vi "sweep(SubVI).vi"(0 "data":refnum<queue>, 1 "类型":enum16{"temp", "field", "position"}(ring), 5 "steps number":i32, 7 "簇":T1={"initialize"=enum."SR830", "6221"={"6221 Resource"="GPIB0::24::INSTR", "Delta status"=FALSE, "电流|RMS(A)"=0.0}, "SR830+6221"={"source"=0, "Current(A)"=0.0, "阻抗(Ohm)"=0.0, "SR830 1"=FALSE, "SR830 2"=FALSE, "SR830 3"=FALSE, "SR830 4"=FALSE, "VISA 1"="", "VISA 2"="", "VISA 3"="", "VISA 4"="", "Reserve 1"=0, "Reserve 2"=-1, "Reserve 3"=-1, "Reserve 4"=-1, "Sensitivity 1"=-1, "Sensitivity 2"=0, "Sensitivity 3"=-1, "Sensitivity 4"=-1, "量程入 1"=0, "量程入 2"=0, "量程入 3"=0, "量程入 4"=0}, "2400"={"2400"=FALSE, "VISA"=""}, "ch"={"ch"=[], "current"=[], "change?"=[], "holding current\nwhen change ch?"=FALSE}, "Instrument"={"335 Resource"="GPIB0::24::INSTR", "Input (0:A)"=0, "Instrument Type"=enum."SVSM", "quantum design"=refnum, "Heater Output (1:1)"=1, "semaphore"=refnum, "TCP master instance"=refnum, "335 Status"=refnum, "M24C Resource"="GPIB0::24::INSTR", "4G supply"="GPIB0::24::INSTR", "Temp Status 24C"=refnum, "Temp"=refnum, "9T信号"=refnum, "limit"={"Field limit"=0.0, "Field rate limit"=0.0, "Temp limit"=0.0, "Temp low limit"=0.0, "Temp rate limit "=0.0}, "4g supply status"=refnum, "vi路径"=""}, "Aborting"=refnum, "数据文件"=refnum, "warning"=refnum, "2614B"={"2614B chA"=FALSE, "2614B chB"=FALSE, "VISA"=""}} {"Instrument"."Input (0:A)" items=["A", "B"]; "Instrument"."Heater Output (1:1)" items=["1"=1, "2"=2]; "SR830+6221"."Sensitivity 4" items=["Auto Gain"=-1, "2 nV/fA"=0, "5 nV/fA"=1, "10 nV/fA"=2, "20 nV/fA"=3, "50 nV/fA"=4, "100 nV/fA"=5, "200 nV/fA"=6, "500 nV/fA"=7, "1 uV/pA"=8, "2 uV/pA"=9, "5 uV/pA"=10, "10 uV/pA"=11, "20 uV/pA"=12, "50 uV/pA"=13, "100 uV/pA"=14, "200 uV/pA"=15, "500 uV/pA"=16, "1 mV/nA"=17, "2 mV/nA"=18, "5 mV/nA"=19, "10 mV/nA"=20, "20 mV/nA"=21, "50 mV/nA"=22, "100 mV/nA"=23, "200 mV/nA"=24, "500 mV/mA"=25, "1 V/uA"=26]; "SR830+6221"."Sensitivity 3" items=["Auto Gain"=-1, "2 nV/fA"=0, "5 nV/fA"=1, "10 nV/fA"=2, "20 nV/fA"=3, "50 nV/fA"=4, "100 nV/fA"=5, "200 nV/fA"=6, "500 nV/fA"=7, "1 uV/pA"=8, "2 uV/pA"=9, "5 uV/pA"=10, "10 uV/pA"=11, "20 uV/pA"=12, "50 uV/pA"=13, "100 uV/pA"=14, "200 uV/pA"=15, "500 uV/pA"=16, "1 mV/nA"=17, "2 mV/nA"=18, "5 mV/nA"=19, "10 mV/nA"=20, "20 mV/nA"=21, "50 mV/nA"=22, "100 mV/nA"=23, "200 mV/nA"=24, "500 mV/mA"=25, "1 V/uA"=26]; "SR830+6221"."Sensitivity 1" items=["Auto Gain"=-1, "2 nV/fA"=0, "5 nV/fA"=1, "10 nV/fA"=2, "20 nV/fA"=3, "50 nV/fA"=4, "100 nV/fA"=5, "200 nV/fA"=6, "500 nV/fA"=7, "1 uV/pA"=8, "2 uV/pA"=9, "5 uV/pA"=10, "10 uV/pA"=11, "20 uV/pA"=12, "50 uV/pA"=13, "100 uV/pA"=14, "200 uV/pA"=15, "500 uV/pA"=16, "1 mV/nA"=17, "2 mV/nA"=18, "5 mV/nA"=19, "10 mV/nA"=20, "20 mV/nA"=21, "50 mV/nA"=22, "100 mV/nA"=23, "200 mV/nA"=24, "500 mV/mA"=25, "1 V/uA"=26]; "SR830+6221"."Sensitivity 2" items=["Auto Gain"=-1, "2 nV/fA"=0, "5 nV/fA"=1, "10 nV/fA"=2, "20 nV/fA"=3, "50 nV/fA"=4, "100 nV/fA"=5, "200 nV/fA"=6, "500 nV/fA"=7, "1 uV/pA"=8, "2 uV/pA"=9, "5 uV/pA"=10, "10 uV/pA"=11, "20 uV/pA"=12, "50 uV/pA"=13, "100 uV/pA"=14, "200 uV/pA"=15, "500 uV/pA"=16, "1 mV/nA"=17, "2 mV/nA"=18, "5 mV/nA"=19, "10 mV/nA"=20, "20 mV/nA"=21, "50 mV/nA"=22, "100 mV/nA"=23, "200 mV/nA"=24, "500 mV/mA"=25, "1 V/uA"=26]; "SR830+6221"."Reserve 4" items=["Auto Gain"=-1, "2 nV/fA"=0, "5 nV/fA"=1, "10 nV/fA"=2, "20 nV/fA"=3, "50 nV/fA"=4, "100 nV/fA"=5, "200 nV/fA"=6, "500 nV/fA"=7, "1 uV/pA"=8, "2 uV/pA"=9, "5 uV/pA"=10, "10 uV/pA"=11, "20 uV/pA"=12, "50 uV/pA"=13, "100 uV/pA"=14, "200 uV/pA"=15, "500 uV/pA"=16, "1 mV/nA"=17, "2 mV/nA"=18, "5 mV/nA"=19, "10 mV/nA"=20, "20 mV/nA"=21, "50 mV/nA"=22, "100 mV/nA"=23, "200 mV/nA"=24, "500 mV/mA"=25, "1 V/uA"=26]; "SR830+6221"."Reserve 3" items=["Auto Reserve"=-1, "High Reserve"=0, "Normal"=1, "Low Noise"=2]; "SR830+6221"."Reserve 2" items=["Auto Reserve"=-1, "High Reserve"=0, "Normal"=1, "Low Noise"=2]; "SR830+6221"."Reserve 1" items=["Auto Reserve"=-1, "High Reserve"=0, "Normal"=1, "Low Noise"=2]; "SR830+6221"."source" items=["SR830 1", "SR830 2", "SR830 3", "SR830 4"]}, 9 "Field":dbl=300.0, 11 "Mode":i32(ring) items=["Persistent", "Driven"], 13 "Field 2":dbl=300.0, 14 "Rate、speed":dbl=10.0) -> (4 "输出簇":T1={"initialize"=enum."SR830", "6221"={"6221 Resource"="GPIB0::24::INSTR", "Delta status"=FALSE, "电流|RMS(A)"=0.0}, "SR830+6221"={"source"=0, "Current(A)"=0.0, "阻抗(Ohm)"=0.0, "SR830 1"=FALSE, "SR830 2"=FALSE, "SR830 3"=FALSE, "SR830 4"=FALSE, "VISA 1"="", "VISA 2"="", "VISA 3"="", "VISA 4"="", "Reserve 1"=0, "Reserve 2"=-1, "Reserve 3"=-1, "Reserve 4"=-1, "Sensitivity 1"=-1, "Sensitivity 2"=0, "Sensitivity 3"=-1, "Sensitivity 4"=-1, "量程入 1"=0, "量程入 2"=0, "量程入 3"=0, "量程入 4"=0}, "2400"={"2400"=FALSE, "VISA"=""}, "ch"={"ch"=[], "current"=[], "change?"=[], "holding current\nwhen change ch?"=FALSE}, "Instrument"={"335 Resource"="GPIB0::24::INSTR", "Input (0:A)"=0, "Instrument Type"=enum."SVSM", "quantum design"=refnum, "Heater Output (1:1)"=1, "semaphore"=refnum, "TCP master instance"=refnum, "335 Status"=refnum, "M24C Resource"="GPIB0::24::INSTR", "4G supply"="GPIB0::24::INSTR", "Temp Status 24C"=refnum, "Temp"=refnum, "9T信号"=refnum, "limit"={"Field limit"=0.0, "Field rate limit"=0.0, "Temp limit"=0.0, "Temp low limit"=0.0, "Temp rate limit "=0.0}, "4g supply status"=refnum, "vi路径"=""}, "Aborting"=refnum, "数据文件"=refnum, "warning"=refnum, "2614B"={"2614B chA"=FALSE, "2614B chB"=FALSE, "VISA"=""}} {"Instrument"."Input (0:A)" items=["A", "B"]; "Instrument"."Heater Output (1:1)" items=["1"=1, "2"=2]; "SR830+6221"."Sensitivity 4" items=["Auto Gain"=-1, "2 nV/fA"=0, "5 nV/fA"=1, "10 nV/fA"=2, "20 nV/fA"=3, "50 nV/fA"=4, "100 nV/fA"=5, "200 nV/fA"=6, "500 nV/fA"=7, "1 uV/pA"=8, "2 uV/pA"=9, "5 uV/pA"=10, "10 uV/pA"=11, "20 uV/pA"=12, "50 uV/pA"=13, "100 uV/pA"=14, "200 uV/pA"=15, "500 uV/pA"=16, "1 mV/nA"=17, "2 mV/nA"=18, "5 mV/nA"=19, "10 mV/nA"=20, "20 mV/nA"=21, "50 mV/nA"=22, "100 mV/nA"=23, "200 mV/nA"=24, "500 mV/mA"=25, "1 V/uA"=26]; "SR830+6221"."Sensitivity 3" items=["Auto Gain"=-1, "2 nV/fA"=0, "5 nV/fA"=1, "10 nV/fA"=2, "20 nV/fA"=3, "50 nV/fA"=4, "100 nV/fA"=5, "200 nV/fA"=6, "500 nV/fA"=7, "1 uV/pA"=8, "2 uV/pA"=9, "5 uV/pA"=10, "10 uV/pA"=11, "20 uV/pA"=12, "50 uV/pA"=13, "100 uV/pA"=14, "200 uV/pA"=15, "500 uV/pA"=16, "1 mV/nA"=17, "2 mV/nA"=18, "5 mV/nA"=19, "10 mV/nA"=20, "20 mV/nA"=21, "50 mV/nA"=22, "100 mV/nA"=23, "200 mV/nA"=24, "500 mV/mA"=25, "1 V/uA"=26]; "SR830+6221"."Sensitivity 1" items=["Auto Gain"=-1, "2 nV/fA"=0, "5 nV/fA"=1, "10 nV/fA"=2, "20 nV/fA"=3, "50 nV/fA"=4, "100 nV/fA"=5, "200 nV/fA"=6, "500 nV/fA"=7, "1 uV/pA"=8, "2 uV/pA"=9, "5 uV/pA"=10, "10 uV/pA"=11, "20 uV/pA"=12, "50 uV/pA"=13, "100 uV/pA"=14, "200 uV/pA"=15, "500 uV/pA"=16, "1 mV/nA"=17, "2 mV/nA"=18, "5 mV/nA"=19, "10 mV/nA"=20, "20 mV/nA"=21, "50 mV/nA"=22, "100 mV/nA"=23, "200 mV/nA"=24, "500 mV/mA"=25, "1 V/uA"=26]; "SR830+6221"."Sensitivity 2" items=["Auto Gain"=-1, "2 nV/fA"=0, "5 nV/fA"=1, "10 nV/fA"=2, "20 nV/fA"=3, "50 nV/fA"=4, "100 nV/fA"=5, "200 nV/fA"=6, "500 nV/fA"=7, "1 uV/pA"=8, "2 uV/pA"=9, "5 uV/pA"=10, "10 uV/pA"=11, "20 uV/pA"=12, "50 uV/pA"=13, "100 uV/pA"=14, "200 uV/pA"=15, "500 uV/pA"=16, "1 mV/nA"=17, "2 mV/nA"=18, "5 mV/nA"=19, "10 mV/nA"=20, "20 mV/nA"=21, "50 mV/nA"=22, "100 mV/nA"=23, "200 mV/nA"=24, "500 mV/mA"=25, "1 V/uA"=26]; "SR830+6221"."Reserve 4" items=["Auto Gain"=-1, "2 nV/fA"=0, "5 nV/fA"=1, "10 nV/fA"=2, "20 nV/fA"=3, "50 nV/fA"=4, "100 nV/fA"=5, "200 nV/fA"=6, "500 nV/fA"=7, "1 uV/pA"=8, "2 uV/pA"=9, "5 uV/pA"=10, "10 uV/pA"=11, "20 uV/pA"=12, "50 uV/pA"=13, "100 uV/pA"=14, "200 uV/pA"=15, "500 uV/pA"=16, "1 mV/nA"=17, "2 mV/nA"=18, "5 mV/nA"=19, "10 mV/nA"=20, "20 mV/nA"=21, "50 mV/nA"=22, "100 mV/nA"=23, "200 mV/nA"=24, "500 mV/mA"=25, "1 V/uA"=26]; "SR830+6221"."Reserve 3" items=["Auto Reserve"=-1, "High Reserve"=0, "Normal"=1, "Low Noise"=2]; "SR830+6221"."Reserve 2" items=["Auto Reserve"=-1, "High Reserve"=0, "Normal"=1, "Low Noise"=2]; "SR830+6221"."Reserve 1" items=["Auto Reserve"=-1, "High Reserve"=0, "Normal"=1, "Low Noise"=2]; "SR830+6221"."source" items=["SR830 1", "SR830 2", "SR830 3", "SR830 4"]}, 8 "错误输出":errorcluster)   [LabVIEW 2019, in "Scan.lvlib"]
uses:
  Scan.lvlib
  ctl/config.ctl
  <vilib>/NI/Modbus Library/API/Master/Modbus Master.lvclass
  ctl/initialize.ctl
  ctl/Instrument.ctl
  ctl/Instrument Type.ctl
  lib/QDInstrument.dll
  ctl/335 state.ctl
  ctl/limit.ctl
  ctl/9T mag field stauts.ctl
  ctl/warning.ctl
  SubVI.lvlib
  User lib.lvlib
  Get value.lvlib
  9T cmag.lvlib
panel:
  out "Field\nStatus 4":i32(ring) items=["MagnetUnknown"=0, "StablePersistent"=1, "WarmingSwitch"=2, "CoolingSwitch"=3, "StableDriven"=4, "Iterating"=5, "Charging"=6, "Discharging"=7, "CurrentError"=8, "MagnetFailure"=15]
  out "Temperature\nStatus 3":i32(ring) items=["TemperatureUnknown"=0, "Stable"=1, "Tracking"=2, "Near"=5, "Chasing"=6, "Filling"=7, "Standby"=10, "Disabled"=13, "ImpedanceNotFunction"=14, "TempFailure"=15]
  out "Temperature\nStatus":i32(ring) items=["TemperatureUnknown"=0, "Stable"=1, "Tracking"=2, "Near"=5, "Chasing"=6, "Filling"=7, "Standby"=10, "Disabled"=13, "ImpedanceNotFunction"=14, "TempFailure"=15]
  out "Field\nStatus 2":i32(ring) items=["MagnetUnknown"=0, "StablePersistent"=1, "WarmingSwitch"=2, "CoolingSwitch"=3, "StableDriven"=4, "Iterating"=5, "Charging"=6, "Discharging"=7, "CurrentError"=8, "MagnetFailure"=15]
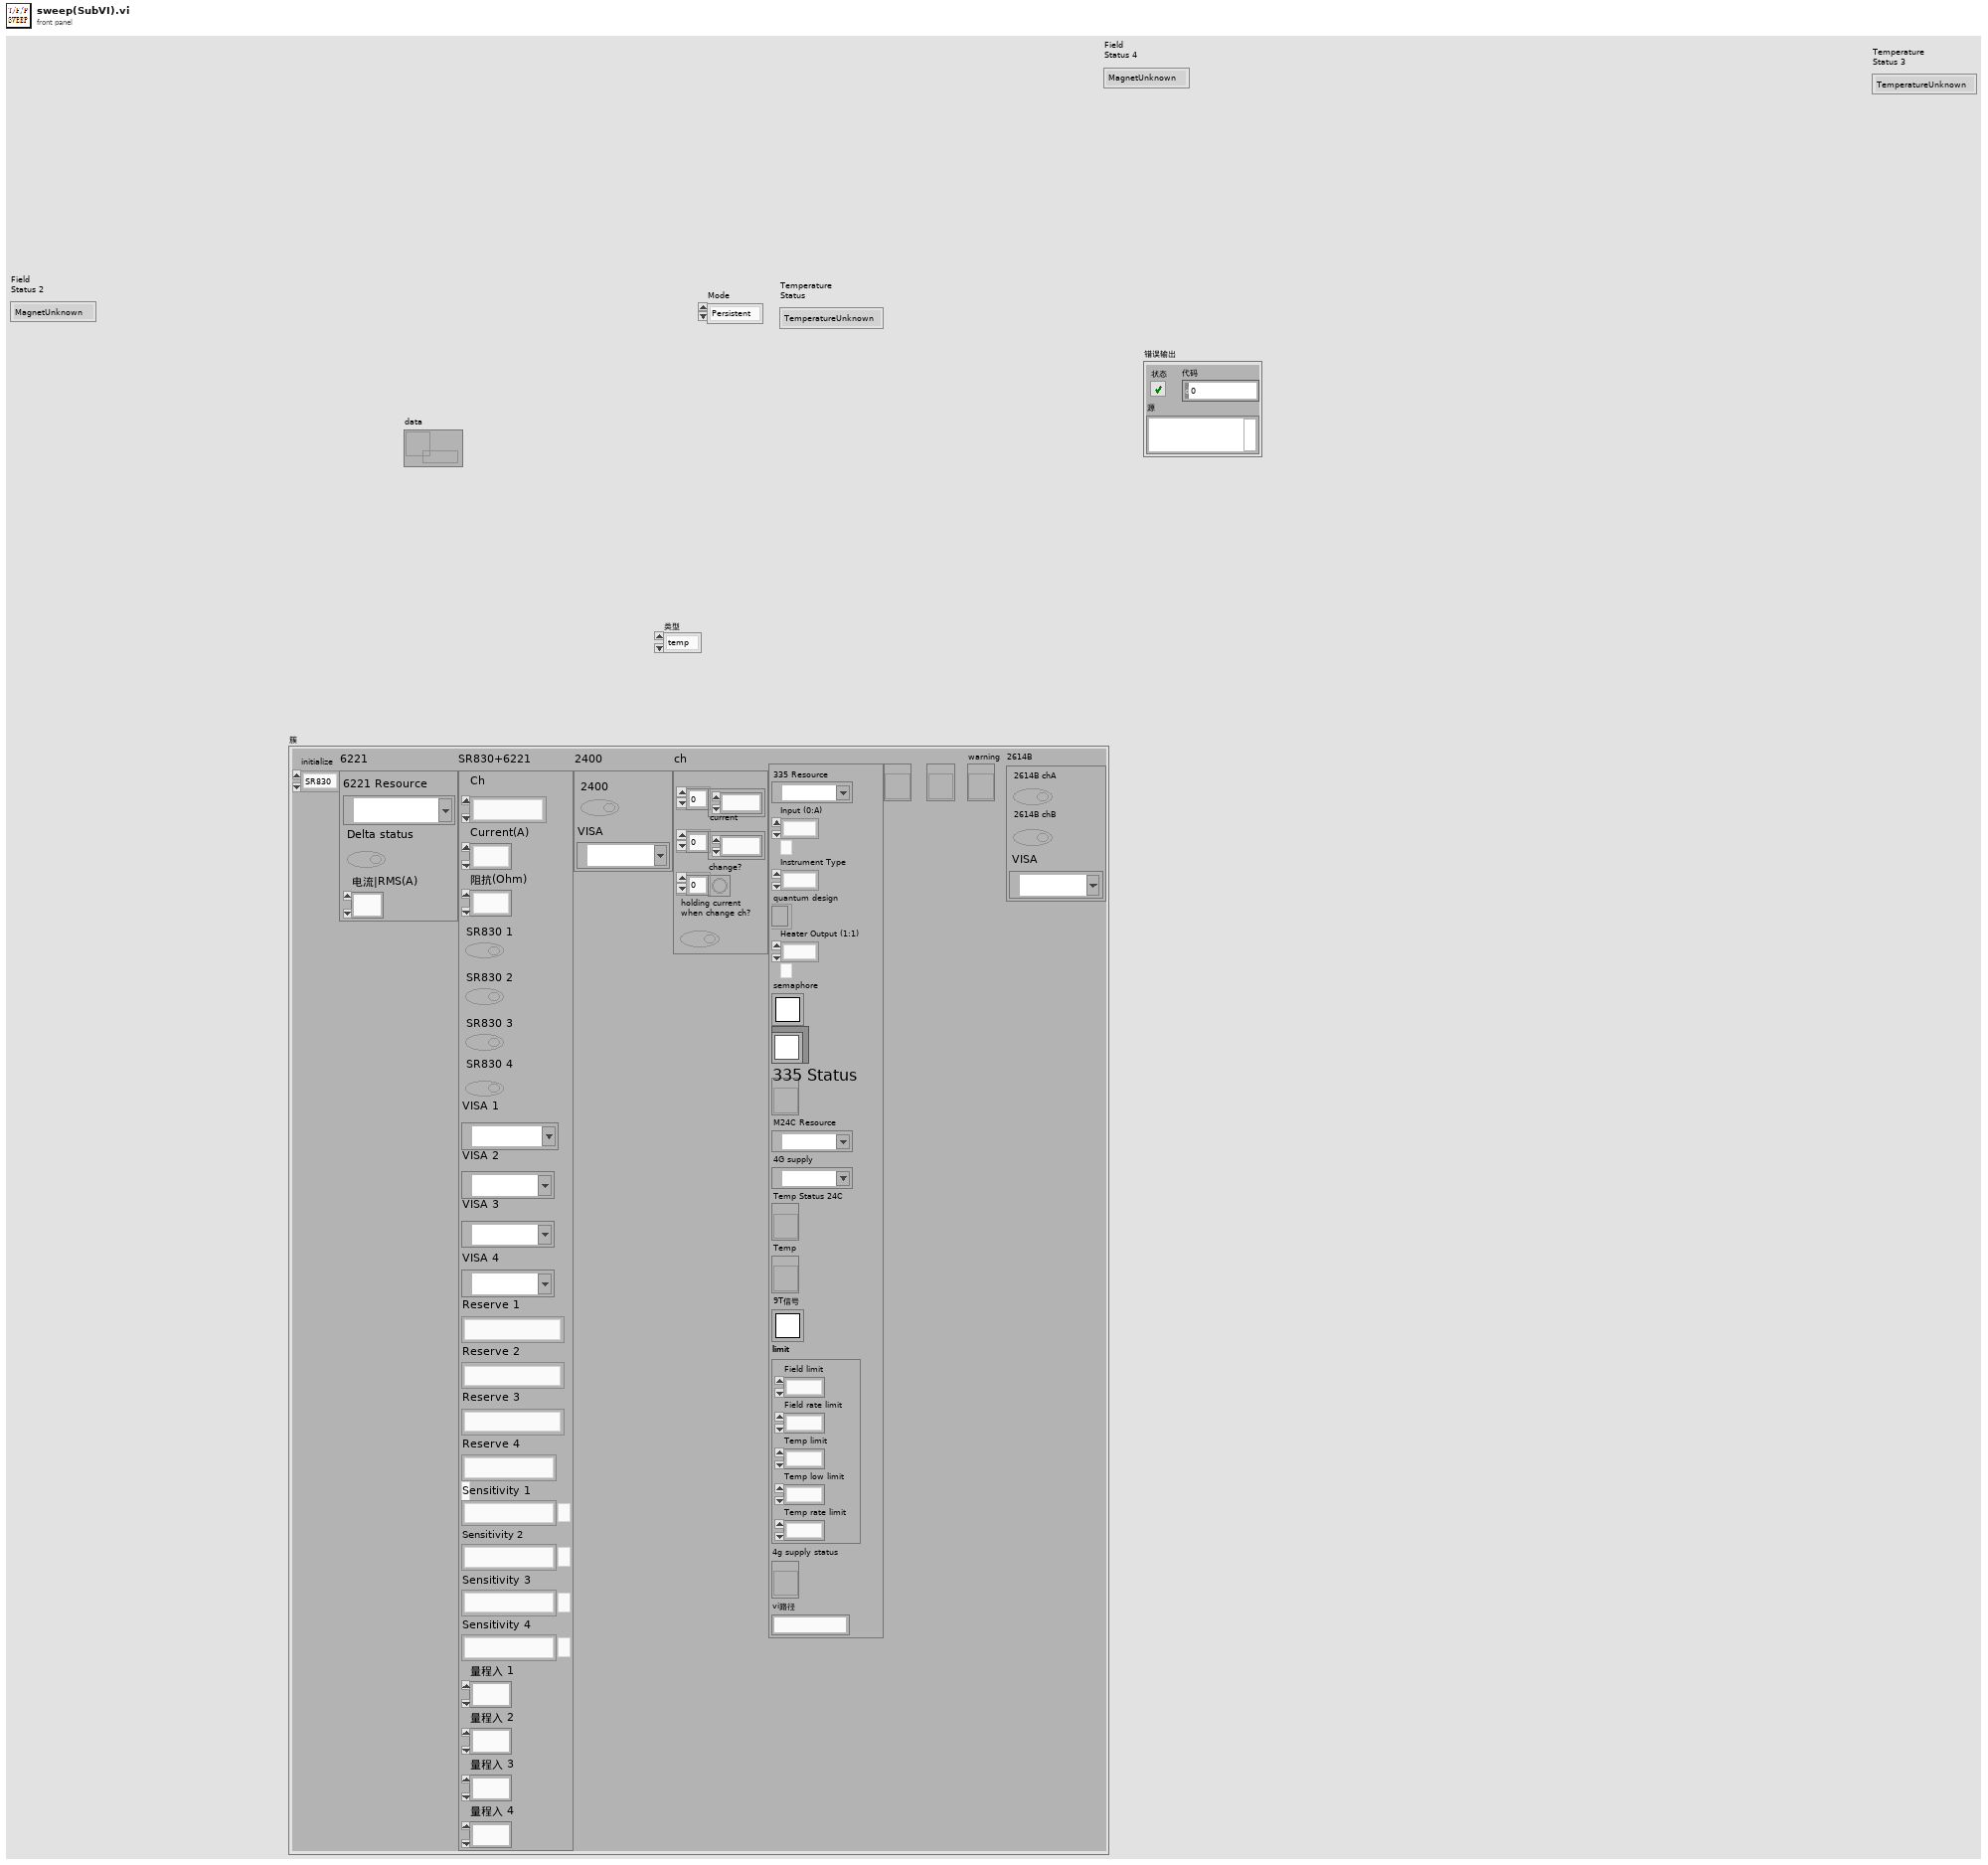
[diagram p1: front panel]
types:
  T1 = typedef "config.ctl" = cluster{"initialize":T2, "6221":cluster{"6221 Resource":refnum<visa-resource-name>, "Delta status":bool, "电流|RMS(A)":dbl}, "SR830+6221":cluster{"source":u16, "Current(A)":dbl, "阻抗(Ohm)":dbl, "SR830 1":bool, "SR830 2":bool, "SR830 3":bool, "SR830 4":bool, "VISA 1":refnum<visa-resource-name>, "VISA 2":refnum<visa-resource-name>, "VISA 3":refnum<visa-resource-name>, "VISA 4":refnum<visa-resource-name>, "Reserve 1":i16, "Reserve 2":i16, "Reserve 3":i16, "Reserve 4":i16, "Sensitivity 1":i16, "Sensitivity 2":i16, "Sensitivity 3":i16, "Sensitivity 4":i16, "量程入 1":i32, "量程入 2":i32, "量程入 3":i32, "量程入 4":i32}, "2400":cluster{"2400":bool, "VISA":refnum<visa-resource-name>}, "ch":cluster{"ch":i32[], "current":dbl[], "change?":bool[], "holding current\nwhen change ch?":bool}, "Instrument":T3, "Aborting":refnum<vi>, "数据文件":refnum<vi>, "warning":refnum<vi>, "2614B":cluster{"2614B chA":bool, "2614B chB":bool, "VISA":refnum<visa-resource-name>}}
  T2 = typedef "initialize.ctl" = enum16{"SR830", "keithley6221-SR830", "Delta", "Delta-tunnelling", "keithley6221-2182-DC"}
  T3 = typedef "Instrument.ctl" = cluster{"335 Resource":refnum<visa-resource-name>, "Input (0:A)":u16, "Instrument Type":T4, "quantum design":refnum<k24>, "Heater Output (1:1)":u16, "semaphore":T5, "TCP master instance":refnum<class "Modbus Master.lvclass">, "335 Status":refnum<vi>, "M24C Resource":refnum<visa-resource-name>, "4G supply":refnum<visa-resource-name>, "Temp Status 24C":refnum<vi>, "Temp":refnum<vi>, "9T信号":T5, "limit":T6, "4g supply status":refnum<vi>, "vi路径":string}
  T4 = typedef "Instrument Type.ctl" = enum16{"PPMS", "VersaLab", "DynaCool", "SVSM", "PPMS-Rotate", "Lakeshore335", "9T mag"}
  T5 = typedef "Semaphore RefNum" = refnum<k1>
  T6 = typedef "limit.ctl" = cluster{"Field limit":dbl, "Field rate limit":dbl, "Temp limit":dbl, "Temp low limit":dbl, "Temp rate limit ":dbl}
  T7 = typedef "335 state.ctl" = u16
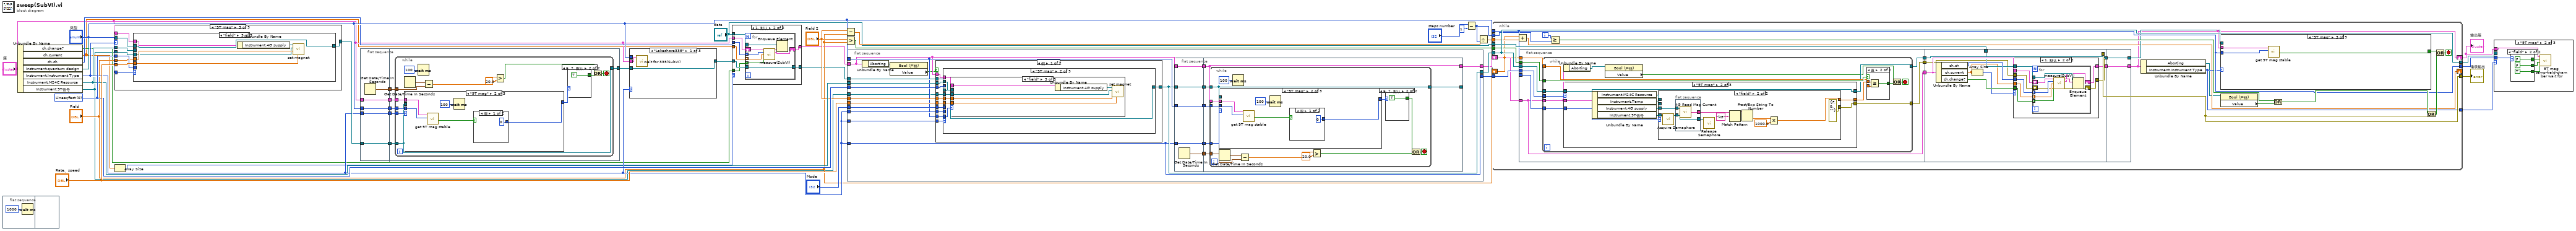
[diagram p0: block diagram]
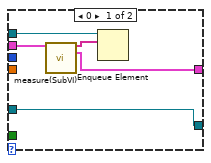
[diagram p2: hidden frame]
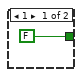
[diagram p3: hidden frame]
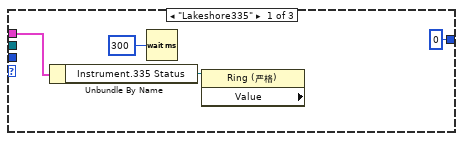
[diagram p4: hidden frame]
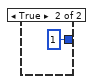
[diagram p5: hidden frame]
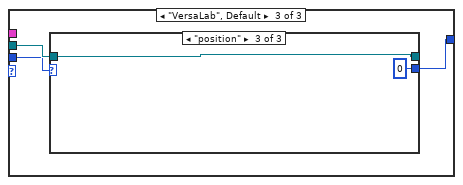
[diagram p6: hidden frame]
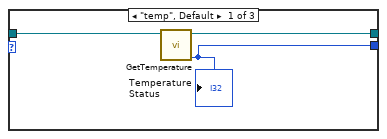
[diagram p7: hidden frame]
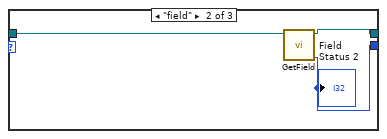
[diagram p8: hidden frame]
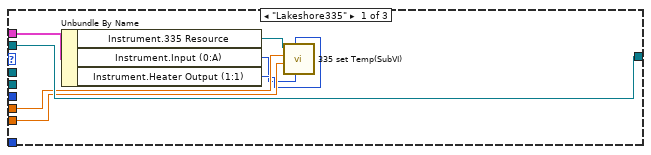
[diagram p9: hidden frame]
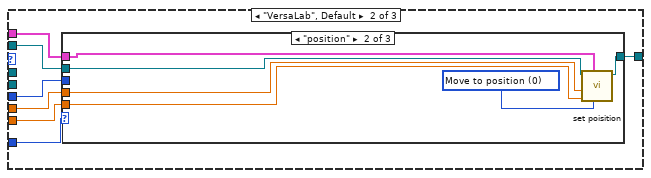
[diagram p10: hidden frame]
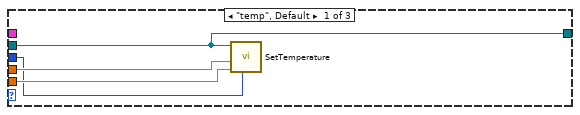
[diagram p11: hidden frame]
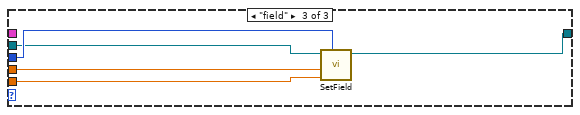
[diagram p12: hidden frame]
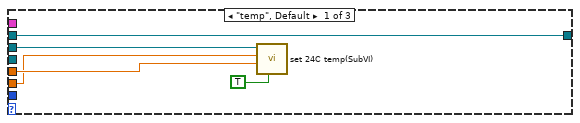
[diagram p13: hidden frame]
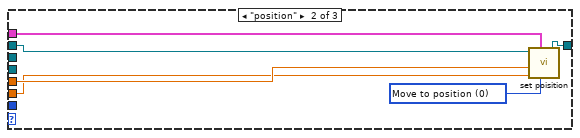
[diagram p14: hidden frame]
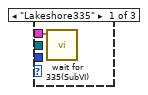
[diagram p15: hidden frame]
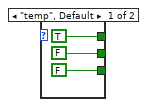
[diagram p16: hidden frame]
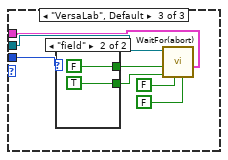
[diagram p17: hidden frame]
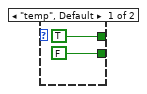
[diagram p18: hidden frame]
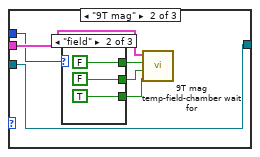
[diagram p19: hidden frame]
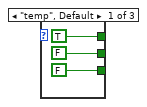
[diagram p20: hidden frame]
diagram:
  w28 = 0 items=["Linear/fast", "NoOvershoot", "Oscillate"] ("Approach")
  n1 = flat-sequence {
    frame #0 {
      n2 = Wait (ms)(milliseconds to wait=u32 1000) -> ()  [unwired: 1 out]
    }
    frame #1 {
    }
  }
  n3 = Unbundle By Name("簇") -> ("ch.change?"=w7:bool[], "ch.current"=w3:dbl[], "ch.ch"=w10:i32[], "Instrument.quantum design"=w27:refnum<k24>, "Instrument.Instrument Type"=w22:T4, "Instrument.M24C Resource"=w21:refnum<visa-resource-name>, "Instrument.9T信号"=w1:T5)
  n4 = case shown="\"9T mag\"" w22 {
    tunnel: "Rate、speed" -> [w45 w55 w79]
    tunnel: [w48 w54 w78] -> w31
    tunnel: "类型" -> [_ w53 w77]
    tunnel: w28 -> [_ w52 w76]
    tunnel: w27 -> [w48 w51 w75]
    tunnel: "Field" -> [w46 w50 w74]
    tunnel: w21 -> [_ _ w73]
    tunnel: "簇" -> [w42 w49 w72]
    tunnel: w1 -> [_ _ w71]
    frame "Lakeshore335" {
      n5 = Unbundle By Name(w42) -> ("Instrument.335 Resource"=w47:refnum<visa-resource-name>, "Instrument.Input (0:A)"=w43:u16, "Instrument.Heater Output (1:1)"=w44:u16)
      n6 = call "335 set Temp(SubVI).vi"("Input (0:A)"=w43, "Output (1:1)"=w44, "Rate"=w45, "Temperature"=w46, "VISA Refnum in"=w47) -> ()  [unwired: 5 in, 2 out]
    }
    frame "VersaLab", Default {
      n7 = case shown="\"position\"" w53 {
        tunnel: w55 -> [w58 w62 w70]
        tunnel: w52 -> [w57 _ w69]
        tunnel: w51 -> [w56 w65 w68]
        tunnel: w50 -> [w59 w63 w67]
        tunnel: [w56 w61 w66] -> w54
        tunnel: w49 -> [_ w60 _]
        frame "temp", Default {
          n8 = call "SetTemperature.vi"("Approach"=w57, "Rate"=w58, "Temperature"=w59, "Instrument Ref In"=w56) -> ()  [unwired: 3 in, 3 out]
        }
        frame "position" {
          w64 = u16 0 items=["Move to position", "Move to limit", "Redefine current position"] ("Mode")
          n9 = call "set poisition.vi"("Mode"=w64, "簇"=w60, "Slow down code\ndefault = 0"=w62, "Position (deg)"=w63, "Instrument Ref In"=w65) -> ("Instrument Ref Out"=w61:refnum<k24>)  [unwired: 3 in, 1 out]
        }
        frame "field" {
          n10 = call "SetField.vi"("Approach"=w69, "Rate"=w70, "Field"=w67, "Instrument Ref In"=w68) -> ("Instrument Ref Out"=w66:refnum<k24>)  [unwired: 3 in, 2 out]
        }
      }
    }
    frame "9T mag" {
      n11 = case shown="\"field\"" w77 {
        tunnel: w79 -> [w81 w87 w92]
        tunnel: w76 -> [_ _ _]
        tunnel: w75 -> [w84 w90 w96]
        tunnel: w74 -> [w82 w88 w93]
        tunnel: [w84 w86 w96] -> w78
        tunnel: w73 -> [w83 _ _]
        tunnel: w72 -> [_ w85 w95]
        tunnel: w71 -> [_ _ w91]
        frame "temp", Default {
          n12 = call "set 24C temp(SubVI).vi"("Control"=TRUE, "Temperature"=w82, "Rate"=w81, "VISA引用句柄输入"=w83) -> ()  [unwired: 7 in, 1 out]
        }
        frame "position" {
          w89 = u16 0 items=["Move to position", "Move to limit", "Redefine current position"] ("Mode")
          n13 = call "set poisition.vi"("Mode"=w89, "簇"=w85, "Slow down code\ndefault = 0"=w87, "Position (deg)"=w88, "Instrument Ref In"=w90) -> ("Instrument Ref Out"=w86:refnum<k24>)  [unwired: 3 in, 1 out]
        }
        frame "field" {
          n14 = Unbundle By Name(w95) -> ("Instrument.4G supply"=w94:refnum<visa-resource-name>)
          n15 = call "set magnet.vi"("Rate(Oe/s)"=w92, "Magnet field(Oe)"=w93, "semaphore"=w91, "VISA Resource Name"=w94) -> ()  [unwired: 5 in, 3 out]
        }
      }
    }
  }
  n16 = Array Size(array=w3) -> (size(s)=w2:i32)
  n17 = flat-sequence {
    tunnel: "簇" -> [w98]
    tunnel: w22 -> [w99]
    tunnel: "类型" -> [w100]
    tunnel: w31 -> [w101]
    tunnel: [w101] -> w20
    tunnel: [w100] -> w19
    tunnel: [w99] -> w18
    tunnel: [w98] -> w17
    tunnel: [w97] -> w16
    tunnel: [w105] -> w26
    tunnel: w20 -> [w107]
    tunnel: w19 -> [w106]
    tunnel: w18 -> [w104]
    tunnel: w17 -> [w103]
    tunnel: w16 -> [w102]
    frame #0 {
      n18 = Get Date/Time In Seconds() -> (seconds since 1Jan1904=w97:timestamp)
    }
    frame #1 {
      n19 = while {
        tunnel: w107 -> [w115]
        tunnel: [w115] -> w105
        tunnel: w106 -> [w120]
        tunnel: w104 -> [w118]
        tunnel: w103 -> [w116]
        tunnel: w102 -> [w111]
        stop <- w108 stop-if-true
        n20 = Get Date/Time In Seconds() -> (seconds since 1Jan1904=w114:timestamp)
        n21 = case shown="\"9T mag\"" w118 {
          tunnel: w115 -> [_ _ w136]
          tunnel: w120 -> [_ w129 w135]
          tunnel: [0 w127 w134] -> w117
          tunnel: w116 -> [w123 w131 _]
          frame "Lakeshore335" {
            n22 = Unbundle By Name(w123) -> ("Instrument.335 Status"=w126:refnum<vi>)
            n23 = Wait (ms)(milliseconds to wait=u32 300) -> ()  [unwired: 1 out]
            n24 = property class="Ring (严格)" props=["Value"](reference=w126) -> ()  [unwired: 1 in, 3 out]
          }
          frame "9T mag" {
            n25 = call "get 9T mag stable.vi"("类型"=w129, "输出簇"=w131) -> ("Stable?"=w128:bool)  [unwired: 9 in]
            n26 = Wait (ms)(milliseconds to wait=u32 100 ("等待时间（毫秒）")) -> ()  [unwired: 1 out]
            n27 = case shown="假" w128 {
              tunnel: [0 ("Field\nStatus") 1 ("Field\nStatus")] -> w127
              frame False {
              }
              frame True {
              }
            }
          }
          frame "VersaLab", Default {
            n28 = case shown="\"position\"" w135 {
              tunnel: w136 -> [w139 w142 w144]
              tunnel: [w137 w141 0 ("Field\nStatus")] -> w134
              tunnel: [w138 w140 w144] -> _
              frame "temp", Default {
                n29 = call "GetTemperature.vi"("Instrument Ref In"=w139) -> ("Temperature\nStatus"=w137:i32, "Instrument Ref Out"=w138:refnum<k24>)  [unwired: 4 in, 3 out]
                "Temperature\nStatus" <- w137
              }
              frame "field" {
                n30 = call "GetField.vi"("Instrument Ref In"=w142) -> ("Field\nStatus"=w141:i32, "Instrument Ref Out"=w140:refnum<k24>)  [unwired: 4 in, 3 out]
                "Field\nStatus 2" <- w141
              }
              frame "position" {
              }
            }
          }
        }
        n31 = Wait (ms)(milliseconds to wait=u32 100) -> ()  [unwired: 1 out]
        n32 = Subtract(x=w114, y=w111) -> (x-y=w113:dbl)
        n33 = Greater?(x=w113, y=20.0) -> (0:w110:bool)
        n34 = case shown="6, 7, 默认" w117 {
          tunnel: [FALSE TRUE] -> w109
          frame 1 {
          }
          frame 6, 7, Default {
          }
        }
        n35 = Or(x=w110, y=w109) -> (x .or. y?=w108:bool)
      }
    }
  }
  n36 = case shown="\"Lakeshore335\"" w22 {
    tunnel: "类型" -> [_ w147 w166]
    tunnel: w26 -> [w146 w152 w164]
    tunnel: [w146 w152 w163] -> w8
    tunnel: "簇" -> [w145 w151 w162]
    frame "Lakeshore335" {
      n37 = call "wait for 335(SubVI).vi"("簇"=w145) -> ()  [unwired: 10 in]
    }
    frame "9T mag" {
      n38 = case shown="\"field\"" w147 {
        tunnel: [TRUE ("temp") FALSE ("temp") FALSE ("temp")] -> w150
        tunnel: [FALSE ("Chamber") FALSE ("Chamber") FALSE ("Chamber")] -> w149
        tunnel: [FALSE ("Field") TRUE ("Field") FALSE ("Field")] -> w148
        frame "temp", Default {
        }
        frame "field" {
        }
        frame "position" {
        }
      }
      n39 = call "9T mag temp-field-chamber wait for.vi"("Field"=w148, "Chamber"=w149, "temp"=w150, "输出簇"=w151) -> ()  [unwired: 8 in]
    }
    frame "VersaLab", Default {
      n40 = case shown="\"field\"" w166 {
        tunnel: [FALSE ("Wait For Field") FALSE ("Wait For Field") TRUE ("Wait For Field")] -> w168
        tunnel: [TRUE ("Wait For Temperature") FALSE ("Wait For Temperature") FALSE ("Wait For Temperature")] -> w167
        tunnel: [FALSE ("Wait For Position") TRUE ("Wait For Position") FALSE ("Wait For Position")] -> w165
        frame "temp", Default {
        }
        frame "position" {
        }
        frame "field" {
        }
      }
      n41 = call "WaitFor(abort).vi"("簇"=w162, "Wait For Chamber"=FALSE, "Wait For Position"=w165, "Wait For Field"=w168, "Wait For Temperature"=w167, "Instrument Ref In"=w164) -> ("Instrument Ref Out"=w163:refnum<k24>)  [unwired: 4 in, 1 out]
    }
  }
  n42 = case shown="1, 默认" w2 {
    tunnel: w10 -> [_ w191]
    tunnel: "簇" -> [w182 w190]
    tunnel: w8 -> [w183 w189]
    tunnel: w7 -> [_ w188]
    tunnel: w3 -> [_ w187]
    tunnel: "data" -> [w180 w186]
    tunnel: [w181 w185] -> w5
    tunnel: [w183 w184] -> w4
    frame 0 {
      n43 = call "measure(SubVI).vi"("config in"=w182) -> ("data"=w179:string[], "config out"=w181:T1)  [unwired: 12 in, 1 out]
      n44 = Enqueue Element(queue=w180, element=w179) -> ()  [unwired: 2 in, 3 out]
    }
    frame 1, Default {
      n45 = for {
        tunnel: w191 -> [w196] mode=indexing
        tunnel: w189 -> [w199]
        tunnel: [w199] -> w184
        tunnel: w188 -> [w194] mode=indexing
        tunnel: w187 -> [w195] mode=indexing
        tunnel: w186 -> [w198]
        shift-right: [w192] -> w185
        shift-left: w190 -> [w197]
        n46 = call "measure(SubVI).vi"("config in"=w197, "ch"=w196, "current"=w195, "change?"=w194) -> ("data"=w193:string[], "config out"=w192:T1)  [unwired: 9 in, 1 out]
        n47 = Enqueue Element(queue=w198, element=w193) -> ()  [unwired: 2 in, 3 out]
      }
    }
  }
  n48 = Subtract(x="Field 2", y="Field") -> (x-y=w40:dbl)
  n49 = Greater?(x="Field 2", y="Field") -> (0:w38:bool)
  n50 = flat-sequence {
    tunnel: [w207] -> w37
    tunnel: w22 -> [w206]
    tunnel: w22 -> [w215]
    tunnel: "类型" -> [w205]
    tunnel: w4 -> [w219]
    tunnel: "Mode" -> [w216]
    tunnel: w28 -> [w220]
    tunnel: "Rate、speed" -> [w218]
    tunnel: "Field 2" -> [w217]
    tunnel: [w206] -> w25
    tunnel: w22 -> [w214]
    tunnel: w21 -> [w213]
    tunnel: w5 -> [w203]
    tunnel: [w204] -> w14
    tunnel: w1 -> [w200]
    frame #0 {
      n51 = Unbundle By Name(w203) -> ("Aborting"=w202:refnum<vi>)
      n52 = property class="Bool (严格)"(reference=w202) -> ("Value"=w201:bool)  [unwired: 1 in, 2 out]
      n53 = case shown="假" w201 {
        tunnel: w220 -> [w232 _]
        tunnel: w219 -> [w231 w281]
        tunnel: w218 -> [w230 _]
        tunnel: w217 -> [w229 _]
        tunnel: w216 -> [w228 _]
        tunnel: w215 -> [w227 _]
        tunnel: w214 -> [w226 _]
        tunnel: w213 -> [w225 _]
        tunnel: [w224 w281] -> w207
        tunnel: w205 -> [w223 _]
        tunnel: w203 -> [w222 _]
        tunnel: w200 -> [w221 _]
        frame False {
          n54 = case shown="\"9T mag\"" w226 {
            tunnel: w223 -> [_ w246 w264]
            tunnel: w232 -> [_ _ w263]
            tunnel: w231 -> [w234 w242 w262]
            tunnel: w230 -> [w235 w243 w261]
            tunnel: w229 -> [w236 w244 w260]
            tunnel: w228 -> [_ _ w259]
            tunnel: w227 -> [_ _ w258]
            tunnel: [w234 w242 w257] -> w224
            tunnel: w225 -> [_ w245 _]
            tunnel: w222 -> [w233 w241 w256]
            tunnel: w221 -> [_ w240 _]
            frame "Lakeshore335" {
              n55 = Unbundle By Name(w233) -> ("Instrument.335 Resource"=w239:refnum<visa-resource-name>, "Instrument.Input (0:A)"=w237:u16, "Instrument.Heater Output (1:1)"=w238:u16)
              n56 = call "335 set Temp(SubVI).vi"("Input (0:A)"=w237, "Output (1:1)"=w238, "Rate"=w235, "Temperature"=w236, "VISA Refnum in"=w239) -> ()  [unwired: 5 in, 2 out]
            }
            frame "9T mag" {
              n57 = case shown="\"field\"" w246 {
                tunnel: w245 -> [w250 _ _]
                tunnel: w244 -> [w249 _ w255]
                tunnel: w243 -> [w248 _ w254]
                tunnel: w241 -> [_ _ w253]
                tunnel: w240 -> [_ _ w251]
                frame "temp", Default {
                  n58 = call "set 24C temp(SubVI).vi"("Control"=TRUE, "Temperature"=w249, "Rate"=w248, "VISA引用句柄输入"=w250) -> ()  [unwired: 7 in, 1 out]
                }
                frame "position" {
                }
                frame "field" {
                  n59 = Unbundle By Name(w253) -> ("Instrument.4G supply"=w252:refnum<visa-resource-name>)
                  n60 = call "set magnet.vi"("Rate(Oe/s)"=w254, "Magnet field(Oe)"=w255, "semaphore"=w251, "VISA Resource Name"=w252) -> ()  [unwired: 5 in, 3 out]
                }
              }
            }
            frame "VersaLab", Default {
              n61 = case shown="\"field\"" w264 {
                tunnel: w261 -> [w267 w271 w280]
                tunnel: w263 -> [w266 _ w279]
                tunnel: w259 -> [_ _ w278]
                tunnel: w262 -> [w265 w273 w277]
                tunnel: w260 -> [w268 w272 w276]
                tunnel: [w265 w274 w275] -> w257
                tunnel: w258 -> [_ _ _]
                tunnel: w256 -> [_ w269 _]
                frame "temp", Default {
                  n62 = call "SetTemperature.vi"("Approach"=w266, "Rate"=w267, "Temperature"=w268, "Instrument Ref In"=w265) -> ()  [unwired: 3 in, 3 out]
                }
                frame "position" {
                  w270 = u16 0 items=["Move to position", "Move to limit", "Redefine current position"] ("Mode")
                  n63 = call "set poisition.vi"("Mode"=w270, "簇"=w269, "Slow down code\ndefault = 0"=w271, "Position (deg)"=w272, "Instrument Ref In"=w273) -> ("Instrument Ref Out"=w274:refnum<k24>)  [unwired: 3 in, 1 out]
                }
                frame "field" {
                  n64 = call "SetField.vi"("Mode"=w278, "Approach"=w279, "Rate"=w280, "Field"=w276, "Instrument Ref In"=w277) -> ("Instrument Ref Out"=w275:refnum<k24>)  [unwired: 2 in, 2 out]
                }
              }
            }
          }
        }
        frame True {
        }
      }
      n65 = flat-sequence {
        tunnel: w203 -> [w283]
        tunnel: w206 -> [w284]
        tunnel: w205 -> [w285]
        tunnel: w207 -> [w286]
        tunnel: [w286] -> w212
        tunnel: [w285] -> w211
        tunnel: [w284] -> w210
        tunnel: [w283] -> w209
        tunnel: [w282] -> w208
        tunnel: [w290] -> _
        tunnel: w212 -> [w292]
        tunnel: w211 -> [w291]
        tunnel: w210 -> [w289]
        tunnel: w209 -> [w287]
        tunnel: w208 -> [w288]
        tunnel: [w287] -> w204
        frame #0 {
          n66 = Get Date/Time In Seconds() -> (seconds since 1Jan1904=w282:timestamp)
        }
        frame #1 {
          n67 = while {
            tunnel: w292 -> [w300]
            tunnel: [w300] -> w290
            tunnel: w291 -> [w305]
            tunnel: w289 -> [w303]
            tunnel: w287 -> [w301]
            tunnel: w288 -> [w293]
            stop <- w294 stop-if-true
            n68 = case shown="\"9T mag\"" w303 {
              tunnel: w300 -> [_ _ w321]
              tunnel: w305 -> [_ w314 w320]
              tunnel: [0 w312 w319] -> w302
              tunnel: w301 -> [w308 w316 _]
              frame "Lakeshore335" {
                n69 = Unbundle By Name(w308) -> ("Instrument.335 Status"=w311:refnum<vi>)
                n70 = Wait (ms)(milliseconds to wait=u32 300) -> ()  [unwired: 1 out]
                n71 = property class="Ring (严格)" props=["Value"](reference=w311) -> ()  [unwired: 1 in, 3 out]
              }
              frame "9T mag" {
                n72 = call "get 9T mag stable.vi"("类型"=w314, "输出簇"=w316) -> ("Stable?"=w313:bool)  [unwired: 9 in]
                n73 = Wait (ms)(milliseconds to wait=u32 100 ("等待时间（毫秒）")) -> ()  [unwired: 1 out]
                n74 = case shown="假" w313 {
                  tunnel: [0 ("Field\nStatus") 1 ("Field\nStatus")] -> w312
                  frame False {
                  }
                  frame True {
                  }
                }
              }
              frame "VersaLab", Default {
                n75 = case shown="\"temp\", 默认" w320 {
                  tunnel: w321 -> [w324 w327 w329]
                  tunnel: [w322 w326 0 ("Field\nStatus")] -> w319
                  tunnel: [w323 w325 w329] -> _
                  frame "temp", Default {
                    n76 = call "GetTemperature.vi"("Instrument Ref In"=w324) -> ("Temperature\nStatus"=w322:i32, "Instrument Ref Out"=w323:refnum<k24>)  [unwired: 4 in, 3 out]
                    "Temperature\nStatus 3" <- w322
                  }
                  frame "field" {
                    n77 = call "GetField.vi"("Instrument Ref In"=w327) -> ("Field\nStatus"=w326:i32, "Instrument Ref Out"=w325:refnum<k24>)  [unwired: 4 in, 3 out]
                    "Field\nStatus 4" <- w326
                  }
                  frame "position" {
                  }
                }
              }
            }
            n78 = Get Date/Time In Seconds() -> (seconds since 1Jan1904=w299:timestamp)
            n79 = Wait (ms)(milliseconds to wait=u32 100) -> ()  [unwired: 1 out]
            n80 = Subtract(x=w299, y=w293) -> (x-y=w298:dbl)
            n81 = Greater?(x=w298, y=20.0) -> (0:w295:bool)
            n82 = case shown="6, 7, 默认" w302 {
              tunnel: [FALSE TRUE] -> w296
              frame 1 {
              }
              frame 6, 7, Default {
              }
            }
            n83 = Or(x=w296, y=w295) -> (x .or. y?=w294:bool)
          }
        }
      }
    }
  }
  n84 = Subtract(x="steps number", y=1) -> (x-y=w32:i32)
  n85 = Divide(x=w40, y=w32) -> (x/y=w11:dbl)
  n86 = while {
    tunnel: w32 -> [w331]
    tunnel: "data" -> [w355]
    tunnel: w37 -> [w353]
    tunnel: w38 -> [w341]
    tunnel: [w353] -> w36
    tunnel: [w351] -> w35
    tunnel: "类型" -> [w345]
    tunnel: [w345] -> w29
    tunnel: w25 -> [w346]
    tunnel: [w342] -> w24
    shift-right: [w340] -> _
    shift-left: "Field" -> [w330]
    shift-right: [w335] -> w13
    shift-left: w14 -> [w339]
    tunnel: w11 -> [w334]
    i -> [w332]
    stop <- w347 stop-if-true
    n87 = Add(x=w330, y=w334) -> (x+y=w340:dbl)
    n88 = flat-sequence {
      tunnel: [w386] -> w356
      tunnel: w353 -> [w389]
      tunnel: w341 -> [w388]
      tunnel: w330 -> [w387]
      tunnel: [w385] -> w352
      tunnel: w345 -> [w384]
      tunnel: w346 -> [w383]
      tunnel: w339 -> [w382]
      tunnel: [w382] -> w338
      tunnel: w356 -> [w467]
      tunnel: w355 -> [w463]
      tunnel: w352 -> [w462]
      tunnel: [w461] -> w351
      tunnel: [w467] -> w349
      tunnel: w338 -> [w466]
      tunnel: [w460] -> w333
      tunnel: [w492] -> w335
      tunnel: [w493] -> w344
      tunnel: w349 -> [w493]
      tunnel: w333 -> [w492]
      frame #0 {
        n89 = while {
          tunnel: w389 -> [w400]
          tunnel: w388 -> [w402]
          tunnel: w387 -> [w401]
          tunnel: [w395] -> w386
          tunnel: [w396] -> w385
          tunnel: w384 -> [w394]
          tunnel: w383 -> [w393]
          tunnel: w382 -> [w390]
          stop <- w397 stop-if-true
          n90 = Unbundle By Name(w390) -> ("Aborting"=w392:refnum<vi>)
          n91 = case shown="\"9T mag\"" w393 {
            selector: w393 -> [_ _ w433]
            tunnel: w400 -> [w406 w411 w438]
            tunnel: [w405 w413 w437] -> w399
            tunnel: [w404 w412 w436] -> w396
            tunnel: [w406 w411 w435] -> w395
            tunnel: w394 -> [_ w415 w434]
            tunnel: w390 -> [w403 w410 _]
            frame "Lakeshore335" {
              n92 = call "Get 335 Main Temp(SubVI).vi"("输入簇"=w403) -> ("error out"=w404:errorcluster, "Main Temp"=w405:dbl)  [unwired: 9 in]
            }
            frame "9T mag" {
              n93 = Unbundle By Name(w410) -> ("Instrument.M24C Resource"=w414:refnum<visa-resource-name>, "Instrument.Temp"=w409:refnum<vi>, "Instrument.4G supply"=w408:refnum<visa-resource-name>, "Instrument.9T信号"=w407:T5)
              n94 = case shown="\"field\"" w415 {
                tunnel: w414 -> [_ _]
                tunnel: [w417 w420] -> w413
                tunnel: [w416 errorcluster {"status"=FALSE, "code"=0, "source"=""} ("error out")] -> w412
                tunnel: w409 -> [w418 _]
                tunnel: w408 -> [_ w426]
                tunnel: w407 -> [_ w419]
                frame "temp", Default {
                  n95 = property class="DigNum (严格)"(reference=w418) -> (error out=w416:errorcluster, "Value"=w417:dbl)  [unwired: 1 in, 1 out]
                }
                frame "field" {
                  n96 = call <vilib>:"Acquire Semaphore.vi"("semaphore"=w419) -> ("semaphore out"=w428:T5)  [unwired: 4 in, 2 out]
                  n97 = flat-sequence {
                    tunnel: [w432] -> w425
                    tunnel: w428 -> [w431]
                    tunnel: [w431] -> w427
                    tunnel: w426 -> [w430]
                    frame #0 {
                      n98 = call "4G Read Mag Current.vi"("VISA session"=w430) -> ("response out"=w432:string)  [unwired: 2 in, 2 out]
                    }
                  }
                  n99 = call <vilib>:"Release Semaphore.vi"("semaphore"=w427) -> ()  [unwired: 5 in, 2 out]
                  n100 = Match Pattern(string=w425, regular expression="kG" ("正则表达式")) -> (before substring=w421:string)  [unwired: 1 in, 3 out]
                  n101 = Fract/Exp String To Number(string=w421) -> (number=w423:dbl)  [unwired: 3 in, 1 out]
                  n102 = Multiply(x=w423, y=1000.0) -> (x*y=w420:dbl)
                }
              }
            }
            frame "VersaLab", Default {
              n103 = case shown="\"temp\", 默认" w434 {
                tunnel: w438 -> [w440 w447 w451]
                tunnel: [w441 w444 w450] -> w437
                tunnel: [w442 w445 w449] -> w436
                tunnel: [w443 w446 w448] -> w435
                tunnel: w433 -> [w439 _ _]
                frame "temp", Default {
                  n104 = call "Get qd Temp (rotate and normal) (SubVI).vi"("Instrument Type"=w439, ".NET引用句柄输入"=w440) -> ()  [unwired: 9 in, 1 out]
                  n105 = call "GetTemperature.vi"("Instrument Ref In"=w440) -> ("Temperature"=w441:dbl, "error out"=w442:errorcluster, "Instrument Ref Out"=w443:refnum<k24>)  [unwired: 4 in, 2 out]
                }
                frame "position" {
                  n106 = call "get poisition.vi"("Instrument Ref In"=w447) -> ("Position"=w444:dbl, "error out"=w445:errorcluster, "Instrument Ref Out 2"=w446:refnum<k24>)  [unwired: 4 in]
                }
                frame "field" {
                  n107 = call "GetField.vi"("Instrument Ref In"=w451) -> ("Field"=w450:dbl, "error out"=w449:errorcluster, "Instrument Ref Out"=w448:refnum<k24>)  [unwired: 4 in, 2 out]
                }
              }
            }
          }
          n108 = property class="Bool (严格)"(reference=w392) -> ("Value"=w391:bool)  [unwired: 1 in, 2 out]
          n109 = case shown="真" w402 {
            tunnel: w399 -> [w454 w457]
            tunnel: w401 -> [w453 w456]
            tunnel: [w452 w455] -> w398
            frame False {
              n110 = Less Or Equal?(x=w454, y=w453) -> (x <= y?=w452:bool)
            }
            frame True {
              n111 = Greater Or Equal?(x=w457, y=w456) -> (x >= y?=w455:bool)
            }
          }
          n112 = Or(x=w391, y=w398) -> (x .or. y?=w397:bool)
        }
      }
      frame #1 {
        n113 = Unbundle By Name(w466) -> ("ch.ch"=w465:i32[], "ch.current"=w459:dbl[], "ch.change?"=w464:bool[])
        n114 = Array Size(array=w459) -> (size(s)=w458:i32)
        n115 = case shown="1, 默认" w458 {
          tunnel: w466 -> [w473 w481]
          tunnel: w465 -> [_ w480]
          tunnel: w459 -> [_ w479]
          tunnel: w464 -> [_ w478]
          tunnel: w463 -> [w468 w477]
          tunnel: w462 -> [w472 w476]
          tunnel: [w471 w475] -> w461
          tunnel: [w470 w474] -> w460
          frame 0 {
            n116 = call "measure(SubVI).vi"("config in"=w473, "error in (no error)"=w472) -> ("data"=w469:string[], "config out"=w470:T1, "error out"=w471:errorcluster)  [unwired: 11 in]
            n117 = Enqueue Element(queue=w468, element=w469) -> ()  [unwired: 2 in, 3 out]
          }
          frame 1, Default {
            n118 = for {
              tunnel: w480 -> [w489] mode=indexing
              tunnel: w478 -> [w487] mode=indexing
              tunnel: w479 -> [w488] mode=indexing
              tunnel: w477 -> [w491]
              shift-right: [w485] -> w474
              shift-left: w481 -> [w490]
              shift-right: [w482] -> w475
              shift-left: w476 -> [w484]
              n119 = call "measure(SubVI).vi"("config in"=w490, "ch"=w489, "current"=w488, "change?"=w487, "error in (no error)"=w484) -> ("data"=w486:string[], "config out"=w485:T1, "error out"=w483:errorcluster)  [unwired: 8 in]
              n120 = Enqueue Element(queue=w491, element=w486, error in (no error)=w483) -> (error out=w482:errorcluster)  [unwired: 1 in, 2 out]
            }
          }
        }
      }
      frame #2 {
      }
    }
    n121 = Greater Or Equal?(x=w332, y=w331) -> (x >= y?=w354:bool)
    n122 = Unbundle By Name(w335) -> ("Aborting"=w337:refnum<vi>, "Instrument.Instrument Type"=w342:T4)
    n123 = case shown="\"9T mag\"" w342 {
      tunnel: w345 -> [w363 _ w379]
      tunnel: w344 -> [w362 _ _]
      tunnel: [w358 w373 w381] -> w343
      tunnel: w335 -> [_ w376 w380]
      frame "PPMS", Default {
        n124 = case shown="\"field\"" w363 {
          tunnel: [FALSE ("WaitForField") FALSE ("WaitForField") TRUE ("WaitForField")] -> w360
          tunnel: [TRUE ("WaitForTemperature") FALSE ("WaitForTemperature") FALSE ("WaitForTemperature")] -> w361
          tunnel: [FALSE ("WaitForPosition") TRUE ("WaitForPosition") FALSE ("WaitForPosition")] -> w359
          frame "temp", Default {
          }
          frame "position" {
          }
          frame "field" {
          }
        }
        n125 = invoke class="QDInstrumentBase" method="WaitConditionReached"(reference=w362, "WaitForTemperature"=w361, "WaitForField"=w360, "WaitForPosition"=w359, "WaitForChamber"=FALSE) -> ("WaitConditionReached"=w358:bool)  [unwired: 2 in, 6 out]
      }
      frame "Lakeshore335" {
        n126 = Unbundle By Name(w376) -> ("Instrument.335 Status"=w375:refnum<vi>)
        n127 = property class="Ring (严格)"(reference=w375) -> ("Value"=w374:T7)  [unwired: 1 in, 2 out]
        n128 = case shown="0, 默认" w374 {
          tunnel: [FALSE TRUE] -> w373
          frame 0, Default {
          }
          frame 1 {
          }
        }
      }
      frame "9T mag" {
        n129 = call "get 9T mag stable.vi"("类型"=w379, "输出簇"=w380) -> ("Stable?"=w381:bool)  [unwired: 9 in]
      }
    }
    n130 = property class="Bool (严格)"(reference=w337) -> ("Value"=w336:bool)  [unwired: 1 in, 2 out]
    n131 = Or(x=w354, y=w336) -> (x .or. y?=w350:bool)
    n132 = Or(x=w350, y=w351) -> (x .or. y?=w348:bool)
    n133 = Or(x=w343, y=w348) -> (x .or. y?=w347:bool)
  }
  "错误输出" <- w35
  "输出簇" <- w13
  n134 = case shown="\"9T mag\"" w24 {
    tunnel: w36 -> [_ _ w508]
    tunnel: w29 -> [_ w496 w507]
    tunnel: w13 -> [w494 w495 w506]
    frame "Lakeshore335" {
      n135 = call "wait for 335(SubVI).vi"("簇"=w494) -> ()  [unwired: 10 in]
    }
    frame "9T mag" {
      n136 = case shown="\"field\"" w496 {
        tunnel: [TRUE ("temp") FALSE ("temp")] -> w499
        tunnel: [FALSE ("Chamber") FALSE ("Chamber")] -> w498
        tunnel: [FALSE ("Field") TRUE ("Field")] -> w497
        frame "temp", Default {
        }
        frame "field" {
        }
      }
      n137 = call "9T mag temp-field-chamber wait for.vi"("Field"=w497, "Chamber"=w498, "temp"=w499, "输出簇"=w495) -> ()  [unwired: 8 in]
    }
    frame "VersaLab", Default {
      n138 = case shown="\"field\"" w507 {
        tunnel: [FALSE ("Wait For Field") TRUE ("Wait For Field")] -> w510
        tunnel: [TRUE ("Wait For Temperature") FALSE ("Wait For Temperature")] -> w509
        frame "temp", Default {
        }
        frame "field" {
        }
      }
      n139 = call "WaitFor(abort).vi"("簇"=w506, "Wait For Chamber"=FALSE, "Wait For Position"=FALSE, "Wait For Field"=w510, "Wait For Temperature"=w509, "Instrument Ref In"=w508) -> ()  [unwired: 4 in, 2 out]
    }
  }
